vi "battery-agent.vi"() -> ()   [LabVIEW 2021]
uses:
  General purpose/MEAS.ctl
  General purpose/REQ.ctl
  General purpose/agent-variables.ctl
  General purpose/daemon-config.ctl
panel:
  out "SCADA Write Error":errorcluster
  in  "SCADA-config":T1={"resource-type"="battery", "SCADA-ip"="192.168.1.2", "SCADA listen-port"=52032}
  in  "daemon-config":T2={"resource-type"="battery", "agent-id"=12, "GA-ip"="192.168.1.1", "GA-port"=52020, "RA-ip"="127.0.0.1", "RA-port"=52001, "listenport-RA-side"=52011, "listenport-GA-side"=52021, "local-ip"="192.168.1.12", "long-term"=FALSE}
  in  "param":T3={"Srated"=25000.0, "eta [pu]"=0.98, "model"={"in-states"={"v1"=0.0, "v2"=0.0, "SoC"=0.0}, "output"={"V"=0.0, "Zeq"=0.0, "Eeq"=0.0}}} {"model"."output"."Eeq" format="%#.6g"; "model"."output"."Zeq" format="%#.6g"; "eta [pu]" format="%#_13g"}
  out "json-adv":string
  out "error out":errorcluster
  in  "ra-res config":T4={"resource-type"="battery", "res-ip"="127.0.0.1", "write-port"=32001, "listen-port"=32011}
  out "wake-up":timestamp
  out "uc":cluster{"Pc":dbl, "Qc":dbl}
  in  "model-dt":u32=100
  in  "SoC_T":dbl=50.0
  out "REQ":T5
  in  "main stop":bool
  out "Meas":T6 {"Ud" format="%#.2f"; "P" format="%#.2f"; "Q" format="%#.2f"}
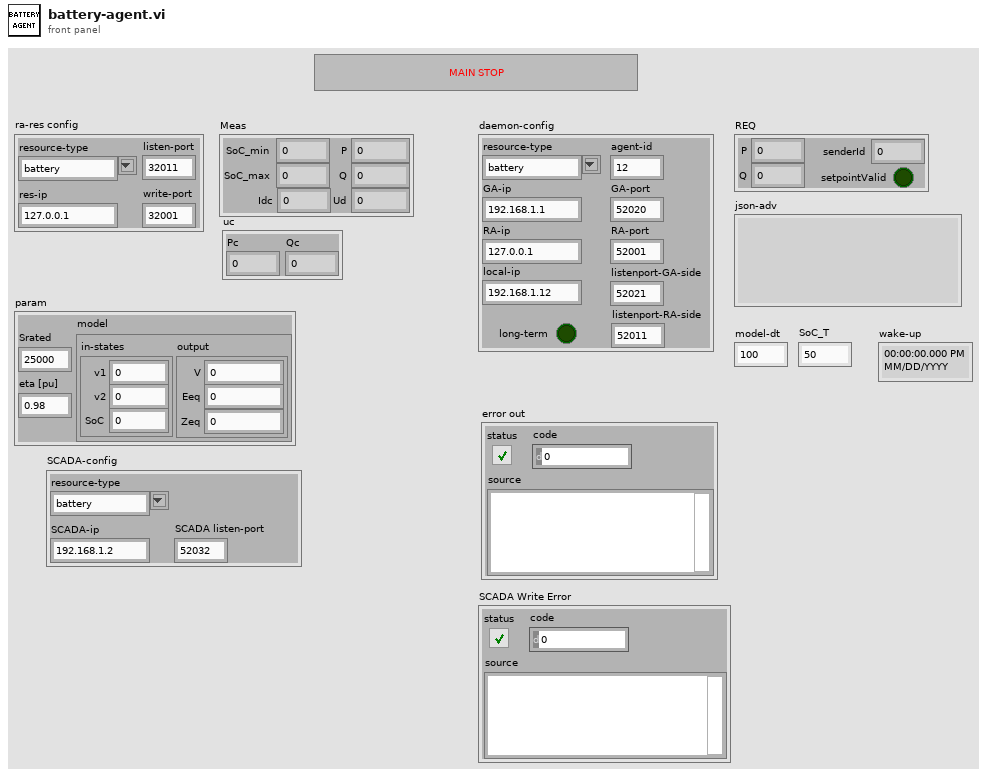
[diagram p1: front panel]
types:
  T1 = cluster{"resource-type":string, "SCADA-ip":string, "SCADA listen-port":u16}
  T2 = typedef "daemon-config.ctl" = cluster{"resource-type":string, "agent-id":u16, "GA-ip":string, "GA-port":u16, "RA-ip":string, "RA-port":u16, "listenport-RA-side":u16, "listenport-GA-side":u16, "local-ip":string, "long-term":bool}
  T3 = typedef "agent-variables.ctl" = cluster{"Srated":dbl, "eta [pu]":dbl, "model":cluster{"in-states":cluster{"v1":dbl, "v2":dbl, "SoC":dbl}, "output":cluster{"V":dbl, "Zeq":dbl, "Eeq":dbl}}}
  T4 = cluster{"resource-type":string, "res-ip":string, "write-port":u16, "listen-port":u16}
  T5 = typedef "REQ.ctl" = cluster{"P":dbl, "Q":dbl, "senderId":u32, "setpointValid":bool}
  T6 = typedef "MEAS.ctl" = cluster{"P":dbl, "Q":dbl, "SoC_max":dbl, "SoC_min":dbl, "Ud":dbl, "Idc":dbl}
  T7 = cluster{"in-states":cluster{"v1":dbl, "v2":dbl, "SoC":dbl}, "output":cluster{"V":dbl, "Zeq":dbl, "Eeq":dbl}}
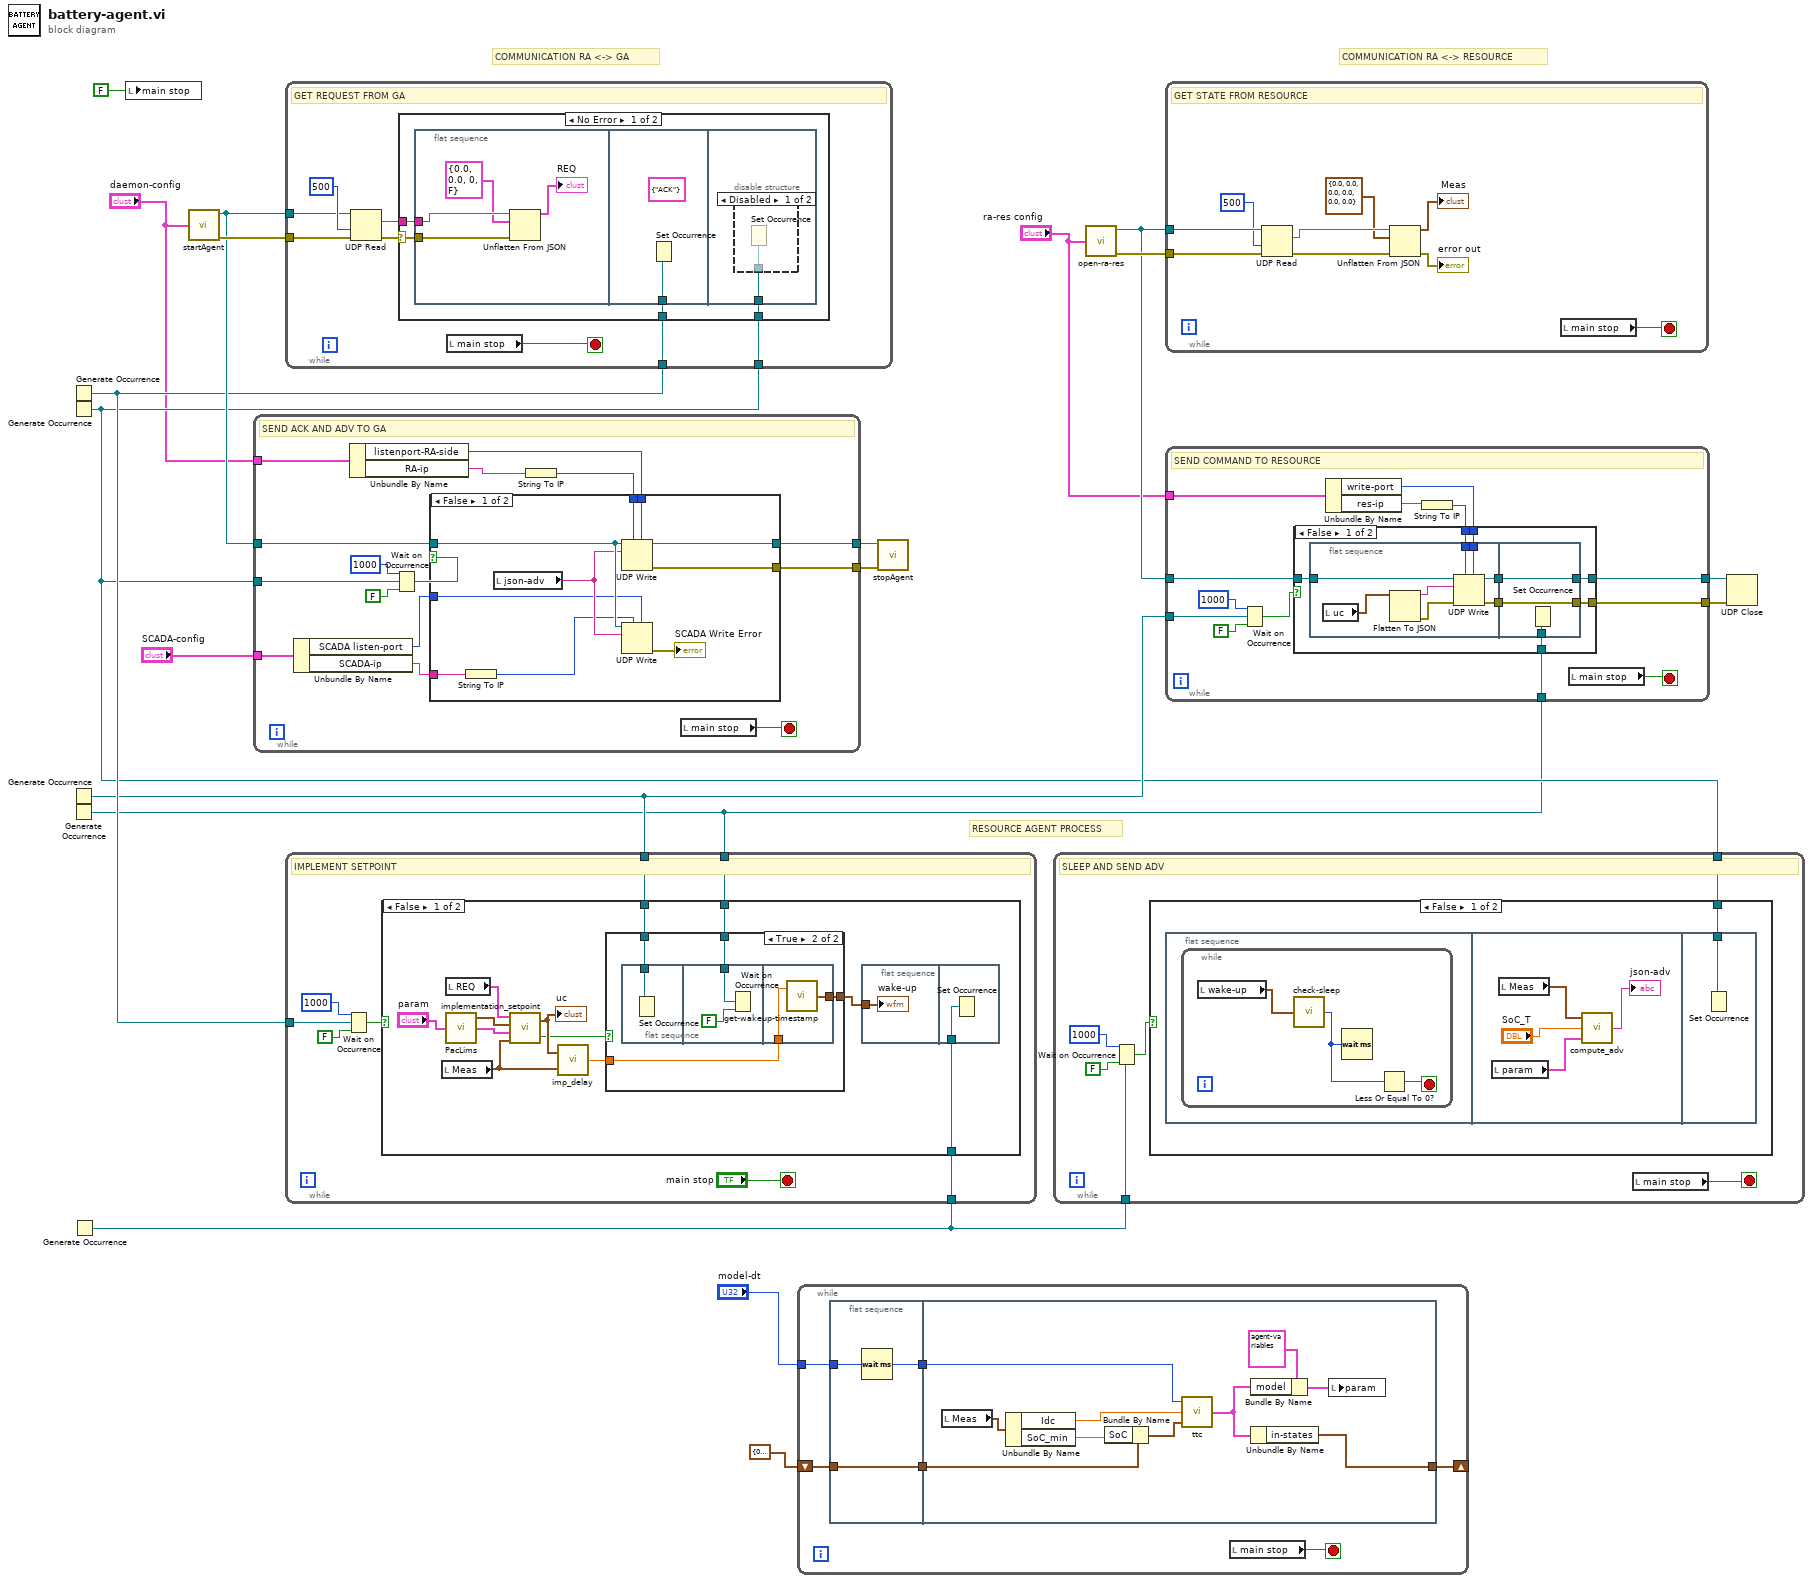
[diagram p0: block diagram]
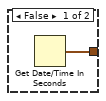
[diagram p2: hidden frame]
diagram:
  # "RESOURCE AGENT PROCESS"
  # "COMMUNICATION RA <-> RESOURCE"
  # "COMMUNICATION RA <-> GA"
  n1 = Generate Occurrence() -> (w15:refnum<k4>)
  n2 = Generate Occurrence() -> (w13:refnum<k4>)
  n3 = Generate Occurrence() -> (w14:refnum<k4>)
  n4 = Generate Occurrence() -> (w12:refnum<k4>)
  n5 = Generate Occurrence() -> (w5:refnum<k4>)
  n6 = local write "main stop"(FALSE ("main stop")) -> ()
  n7 = call "startAgent.vi"("daemon-config"="daemon-config") -> ("error out"=w19:errorcluster, "connection ID"=w16:refnum<k16>)  [unwired: 6 in]
  n8 = while {
    tunnel: [w33] -> w18
    tunnel: [w32] -> w17
    tunnel: "daemon-config" -> [w30]
    tunnel: w13 -> [w27]
    tunnel: w16 -> [w26]
    tunnel: "SCADA-config" -> [w22]
    stop <- w34 stop-if-true
    # "SEND ACK AND ADV TO GA"
    n9 = Unbundle By Name(w22) -> ("SCADA listen-port"=w20:u16, "SCADA-ip"=w21:string)
    n10 = Unbundle By Name(w30) -> ("listenport-RA-side"=w28:u16, "RA-ip"=w31:string)
    n11 = Wait on Occurrence(1:FALSE ("ignore previous (T)"), 2:w27, 3:1000 ("ms timeout (-1)")) -> (0:w25:bool)
    n12 = String To IP(1:w31) -> (0:w29:u32)
    n13 = case shown="False" w25 {
      tunnel: [w44 w45] -> w33
      tunnel: [w43 _] -> w32
      tunnel: w29 -> [w42 _]
      tunnel: w28 -> [w41 _]
      tunnel: w26 -> [w40 w45]
      tunnel: w21 -> [w38 _]
      tunnel: w20 -> [w36 _]
      frame False {
        n14 = String To IP(1:w38) -> (0:w37:u32)
        n15 = local read "json-adv"() -> (w39:string)
        n16 = UDP Write(address=w42, port or service name=w41, connection ID=w40, data in=w39) -> (error out=w43:errorcluster, 3:w44:refnum<k16>)  [unwired: 2 in]
        n17 = UDP Write(address=w37, port or service name=w36, connection ID=w40, data in=w39) -> (error out=→"SCADA Write Error":errorcluster)  [unwired: 2 in, 1 out]
      }
      frame True {
      }
    }
    n18 = local read "main stop"() -> (w34:bool)
  }
  n19 = while {
    tunnel: w16 -> [w49]
    tunnel: w19 -> [w48]
    tunnel: w15 -> [w52]
    tunnel: w13 -> [w51]
    stop <- w53 stop-if-true
    # "GET REQUEST FROM GA"
    n20 = UDP Read(connection ID=w49, timeout ms (25000)=500, 8:w48) -> (data out=w46:string, error out=w47:errorcluster)  [unwired: 4 out]
    n21 = case shown="No Error" w47 {
      selector: w47 -> [w55 _]
      tunnel: w52 -> [w57 _]
      tunnel: w51 -> [w56 _]
      tunnel: w46 -> [w54 _]
      frame No Error {
        n22 = flat-sequence {
          tunnel: w55 -> [w60]
          tunnel: w54 -> [w59]
          tunnel: w57 -> [w62]
          tunnel: w56 -> [w63]
          frame #0 {
            n23 = Unflatten From JSON(JSON string=w59, type and defaults=T5 {"P"=0.0, "Q"=0.0, "senderId"=0, "setpointValid"=FALSE} ("REQ"), error in (no error)=w60) -> (value=→"REQ":T5)  [unwired: 4 in, 1 out]
          }
          frame #1 {
            (unwired) cluster{string} {"ACK"} ("anything")
            n24 = Set Occurrence(w62) -> ()
          }
          frame #2 {
            n25 = disable-structure shown="Disabled" {
              disable-tunnel: w63 -> [w64 _]
              frame Disabled {
                n26 = Set Occurrence(w64) -> ()
              }
              frame Enabled {
              }
            }
          }
        }
      }
      frame Error {
      }
    }
    n27 = local read "main stop"() -> (w53:bool)
  }
  n28 = while {
    tunnel: w15 -> [w66]
    tunnel: w14 -> [w72]
    tunnel: w12 -> [w70]
    tunnel: w5 -> [w69]
    stop <- "main stop" stop-if-true
    # "IMPLEMENT SETPOINT"
    n29 = Wait on Occurrence(1:FALSE ("ignore previous (T)"), 2:w66, 3:1000 ("ms timeout (-1)")) -> (0:w68:bool)
    n30 = case shown="False" w68 {
      tunnel: w72 -> [w84 _]
      tunnel: w70 -> [w83 _]
      tunnel: w69 -> [w74 _]
      frame False {
        n31 = local read "Meas"() -> (w78:T6)
        n32 = local read "REQ"() -> (w80:T5)
        n33 = call "PacLims.vi"("param (in)"="param") -> ("PacLims"=w82:cluster{"Pmax":dbl, "Pmin":dbl}, "param (out)"=w81:T3)  [unwired: 1 out]
        n34 = call "implementation_setpoint.vi"("Meas"=w78, "param"=w81, "PacLims (in)"=w82, "REQ"=w80) -> ("send_cmd?"=w77:bool, "uc"=w79:cluster{"Pc":dbl, "Qc":dbl})
        "uc" <- w79
        n35 = call "imp_delay.vi"("Meas"=w78, "uc"=w79) -> ("res-dt"=w76:dbl)
        n36 = case shown="True" w77 {
          tunnel: w84 -> [_ w91]
          tunnel: w83 -> [_ w90]
          tunnel: w76 -> [_ w89]
          tunnel: [w87 w88] -> w75
          frame False {
            n37 = Get Date/Time In Seconds() -> (seconds since 1Jan1904=w87:timestamp)
          }
          frame True {
            n38 = flat-sequence {
              tunnel: w91 -> [w92]
              tunnel: w90 -> [w94]
              tunnel: w89 -> [w96]
              tunnel: [w95] -> w88
              frame #0 {
                n39 = Set Occurrence(w92) -> ()
              }
              frame #1 {
                n40 = Wait on Occurrence(1:FALSE ("ignore previous (T)"), 2:w94) -> ()  [unwired: 1 in, 1 out]
              }
              frame #2 {
                n41 = call "get-wakeup-timestamp.vi"("Tra"=w96) -> ("wake-up timestamp"=w95:timestamp)  [unwired: 1 in]
              }
            }
          }
        }
        n42 = flat-sequence {
          tunnel: w75 -> [w85]
          tunnel: w74 -> [w86]
          frame #0 {
            "wake-up" <- w85
          }
          frame #1 {
            n43 = Set Occurrence(w86) -> ()
          }
        }
      }
      frame True {
      }
    }
  }
  n44 = while {
    tunnel: "model-dt" -> [w101]
    shift-right: [w99] -> _
    shift-left: cluster{"v1":dbl, "v2":dbl, "SoC":dbl} {"v1"=0.0, "v2"=0.0, "SoC"=0.0} ("in-states") -> [w97]
    stop <- w102 stop-if-true
    n45 = flat-sequence {
      tunnel: w101 -> [w105]
      tunnel: [w104] -> w100
      tunnel: [w103] -> w98
      tunnel: w97 -> [w103]
      tunnel: w100 -> [w114]
      tunnel: [w110] -> w99
      tunnel: w98 -> [w108]
      frame #0 {
        n46 = Wait (ms)(milliseconds to wait=w105) -> (millisecond timer value=w104:u32)
      }
      frame #1 {
        n47 = local read "Meas"() -> (w115:T6)
        n48 = Unbundle By Name(w115) -> ("Idc"=w113:dbl, "SoC_min"=w106:dbl)
        n49 = Bundle By Name(cluster=w108, "SoC"=w106) -> (w107:cluster{"v1":dbl, "v2":dbl, "SoC":dbl})
        n50 = call "ttc.vi"("x[k-1]"=w107, "I"=w113, "Period"=w114) -> ("model"=w109:T7)  [unwired: 2 in]
        n51 = Bundle By Name(cluster=T3 {"Srated"=25000.0, "eta [pu]"=0.98, "model"={"in-states"={"v1"=0.0, "v2"=0.0, "SoC"=0.0}, "output"={"V"=0.0, "Zeq"=0.0, "Eeq"=0.0}}} ("param"), "model"=w109) -> (w112:T3)
        n52 = Unbundle By Name(w109) -> ("in-states"=w110:cluster{"v1":dbl, "v2":dbl, "SoC":dbl})
        n53 = local write "param"(w112) -> ()
      }
    }
    n54 = local read "main stop"() -> (w102:bool)
  }
  n55 = call "stopAgent.vi"("error in"=w17, "connection ID"=w18) -> ()  [unwired: 10 in]
  n56 = while {
    tunnel: w5 -> [w118]
    tunnel: w13 -> [w120]
    stop <- w121 stop-if-true
    # "SLEEP AND SEND ADV"
    n57 = Wait on Occurrence(1:FALSE ("ignore previous (T)"), 2:w118, 3:1000 ("ms timeout (-1)")) -> (0:w119:bool)
    n58 = case shown="False" w119 {
      tunnel: w120 -> [w122 _]
      frame False {
        n59 = flat-sequence {
          tunnel: w122 -> [w130]
          frame #0 {
            n60 = while {
              stop <- w124 stop-if-true
              n61 = local read "wake-up"() -> (w125:timestamp)
              n62 = call "check-sleep.vi"("wake-up timestamp"=w125) -> ("dt"=w123:u32)
              n63 = Wait (ms)(milliseconds to wait=w123) -> ()  [unwired: 1 out]
              n64 = Less Or Equal To 0?(x=w123) -> (x <= 0?=w124:bool)
            }
          }
          frame #1 {
            n65 = local read "param"() -> (w129:T3)
            n66 = local read "Meas"() -> (w128:T6)
            n67 = call "compute_adv.vi"("param"=w129, "SoC_T"="SoC_T", "Meas"=w128) -> ("json-adv"=→"json-adv":string)
          }
          frame #2 {
            n68 = Set Occurrence(w130) -> ()
          }
        }
      }
      frame True {
      }
    }
    n69 = local read "main stop"() -> (w121:bool)
  }
  n70 = call "open-ra-res.vi"("config"="ra-res config") -> ("error out"=w11:errorcluster, "connection ID"=w10:refnum<k16>)  [unwired: 6 in]
  n71 = while {
    tunnel: w10 -> [w138]
    tunnel: w11 -> [w137]
    stop <- w139 stop-if-true
    # "GET STATE FROM RESOURCE"
    n72 = UDP Read(connection ID=w138, timeout ms (25000)=500, 8:w137) -> (data out=w135:string, error out=w134:errorcluster)  [unwired: 4 out]
    n73 = Unflatten From JSON(JSON string=w135, type and defaults=T6 {"P"=0.0, "Q"=0.0, "SoC_max"=0.0, "SoC_min"=0.0, "Ud"=0.0, "Idc"=0.0} ("Meas"), error in (no error)=w134) -> (value=→"Meas":T6, error out=→"error out":errorcluster)  [unwired: 4 in]
    n74 = local read "main stop"() -> (w139:bool)
  }
  n75 = while {
    tunnel: [w151] -> w9
    tunnel: [w150] -> w8
    tunnel: w14 -> [w144]
    tunnel: w10 -> [w149]
    tunnel: w12 -> [w141]
    tunnel: "ra-res config" -> [w148]
    stop <- w152 stop-if-true
    # "SEND COMMAND TO RESOURCE"
    n76 = Wait on Occurrence(1:FALSE ("ignore previous (T)"), 2:w144, 3:1000 ("ms timeout (-1)")) -> (0:w142:bool)
    n77 = Unbundle By Name(w148) -> ("write-port"=w145:u16, "res-ip"=w147:string)
    n78 = String To IP(1:w147) -> (0:w146:u32)
    n79 = case shown="False" w142 {
      tunnel: [w160 w172] -> w151
      tunnel: [w159 _] -> w150
      tunnel: w149 -> [w158 w172]
      tunnel: w146 -> [w157 _]
      tunnel: w145 -> [w156 _]
      tunnel: w141 -> [w153 _]
      frame False {
        n80 = flat-sequence {
          tunnel: w158 -> [w166]
          tunnel: w157 -> [w165]
          tunnel: w156 -> [w164]
          tunnel: [w168] -> w155
          tunnel: [w167] -> w154
          tunnel: [w170] -> w159
          tunnel: [w171] -> w160
          tunnel: w155 -> [w171]
          tunnel: w154 -> [w170]
          tunnel: w153 -> [w169]
          frame #0 {
            n81 = local read "uc"() -> (w161:cluster{"Pc":dbl, "Qc":dbl})
            n82 = Flatten To JSON(anything=w161) -> (JSON string=w162:string, 11:w163:errorcluster)  [unwired: 2 in]
            n83 = UDP Write(address=w165, port or service name=w164, connection ID=w166, data in=w162, 8:w163) -> (error out=w167:errorcluster, 3:w168:refnum<k16>)  [unwired: 1 in]
          }
          frame #1 {
            n84 = Set Occurrence(w169) -> ()
          }
        }
      }
      frame True {
      }
    }
    n85 = local read "main stop"() -> (w152:bool)
  }
  n86 = UDP Close(connection ID=w9, 8:w8) -> ()  [unwired: 2 out]
